vi "Create Manager.Text (Async).vi"(4 "read timeput (ms)":i32=100, 5 "ConfigManager.Text":refnum<class "ConfigManager.Text.lvclass">, 6 "pre-load from disk (T)":bool=TRUE, 7 "Manager.Text Configuration":T1, 8 "error in (no error)":errorcluster, 9 "write delay (ms)":i32, 11 "filepath":path) -> (0 "error out":errorcluster, 3 "ConfigManager.Text out":refnum<class "ConfigManager.Text.lvclass">)   [LabVIEW 2013, in "CfgManager.Text.lvlib" / "ConfigManager.Text.lvclass"]
uses:
  ConfigManager.Text.lvclass
  Configuration -- Cluster.ctl
  FileHeader/FileHeader.lvclass
  FileSignature/FileSignature.lvclass
  ConfigManager.Text.lvclass/ConfigManager.Text.ctl
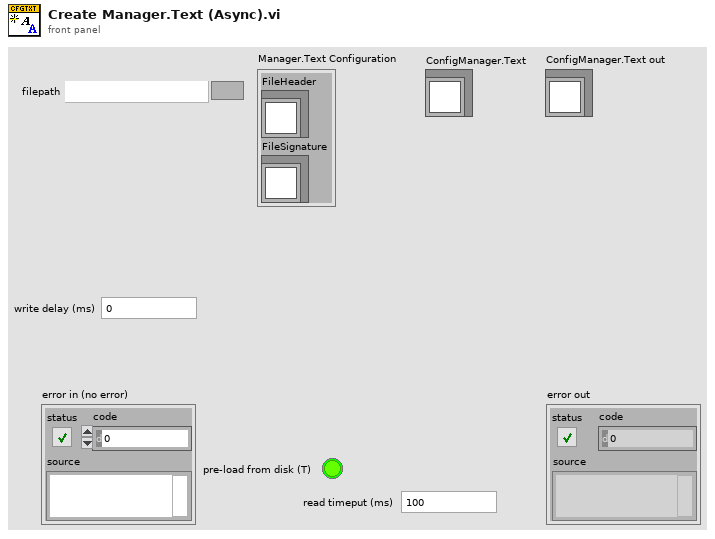
[diagram p1: front panel]
types:
  T1 = typedef "CfgManager.Text.lvlib/ConfigManager.Text.lvclass/Configuration -- Cluster.ctl" = cluster{"FileHeader":refnum<class "FileHeader.lvclass">, "FileSignature":refnum<class "FileSignature.lvclass">}
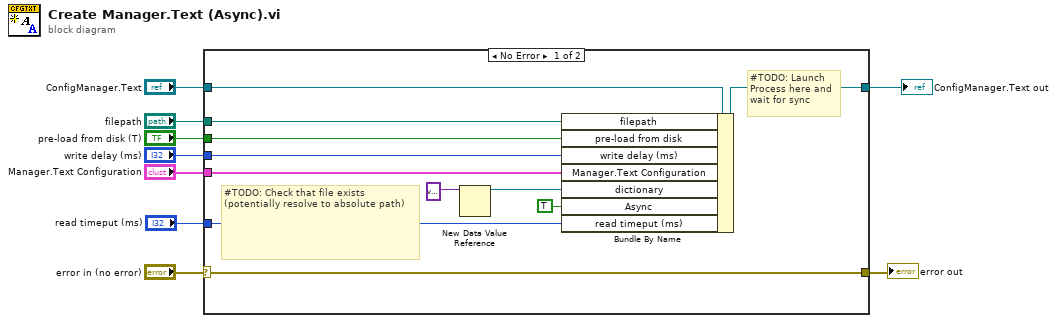
[diagram p0: block diagram]
diagram:
  n1 = case shown="No Error" "error in (no error)" {
    selector: "error in (no error)" -> [w15 w21]
    tunnel: "ConfigManager.Text" -> [w20 w22]
    tunnel: [w19 w22] -> w8
    tunnel: "filepath" -> [w18 _]
    tunnel: "pre-load from disk (T)" -> [w17 _]
    tunnel: "write delay (ms)" -> [w16 _]
    tunnel: [w15 w21] -> w3
    tunnel: "Manager.Text Configuration" -> [w14 _]
    tunnel: "read timeput (ms)" -> [w10 _]
    frame No Error {
      # "#TODO: Launch\nProcess here and\nwait for sync"
      # "#TODO: Check that file exists (potentially resolve to absolute path)"
      n2 = New Data Value Reference(data value=variant ("Variant")) -> (data value reference=w12:refnum<data-value>)  [unwired: 1 in, 1 out]
      n3 = Bundle By Name(cluster=w20, "filepath"=w18, "pre-load from disk"=w17, "write delay (ms)"=w16, "Manager.Text Configuration"=w14, "dictionary"=w12, "Async"=TRUE, "read timeput (ms)"=w10) -> (w19:refnum<class "ConfigManager.Text.lvclass">)
    }
    frame Error {
    }
  }
  "ConfigManager.Text out" <- w8
  "error out" <- w3
